vi "Configure Bridge Resistance.vi"(8 "error in (no error)":errorcluster, 9 "Use Rmeas or Ruser (0: Rmeas(System Default Value))":i32(ring) items=["Rmeas(System Default Value)", "Ruser(User Defined Value)"], 10 "Select Bridge Resistance (1: 200Ohm)":i32(ring)=1 items=["100Ohm", "200Ohm", "300Ohm", "400Ohm"], 11 "VISA resource name":refnum<visa-resource-name>) -> (0 "error out":errorcluster, 3 "VISA resource name out":refnum<visa-resource-name>)   [LabVIEW 2011, in "Agilent N432A.lvlib"]
doc: "Specifies the type and value of the bridge resistance for the thermistor sensor. When Rmeas(system default value) is selected, an externally measured bridge resistance value stored in EEPROM will be used. When Ruser(user difined value) is selected, you can enter a resistance value to be used in power measurement."
uses:
  <instrlib>/Agilent N432A/Agilent N432A.lvlib
panel:
  in  "Ruser Value(100 Ohm)":dbl=100.0
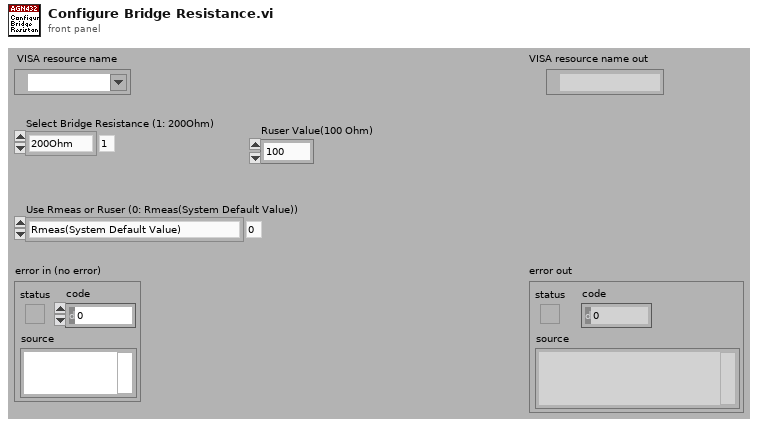
[diagram p1: front panel]
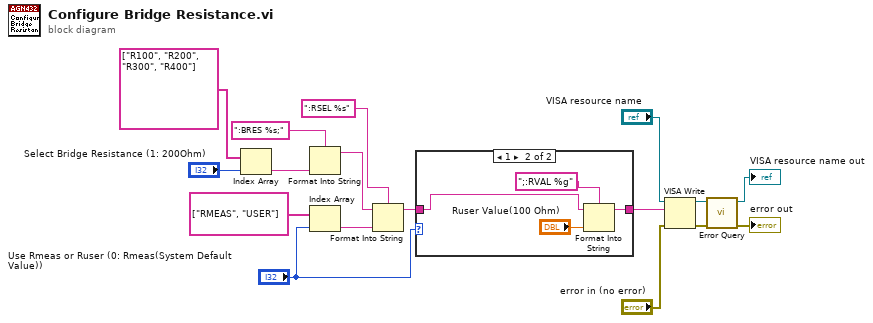
[diagram p0: block diagram]
diagram:
  n1 = Index Array(array=string[] ["R100", "R200", "R300", "R400"], index="Select Bridge Resistance (1: 200Ohm)") -> (element=w6:string)
  n2 = Format Into String(format string=":BRES %s;", w6) -> (resulting string=w3:string)  [unwired: 2 in, 1 out]
  n3 = Index Array(array=string[] ["RMEAS", "USER"], index="Use Rmeas or Ruser (0: Rmeas(System Default Value))") -> (element=w4:string)
  n4 = Format Into String(format string=":RSEL %s", initial string=w3, w4) -> (resulting string=w2:string)  [unwired: 1 in, 1 out]
  n5 = case shown="1" "Use Rmeas or Ruser (0: Rmeas(System Default Value))" {
    tunnel: w2 -> [w18 w20]
    tunnel: [w18 w19] -> w1
    frame 0, Default {
    }
    frame 1 {
      n6 = Format Into String(format string=";:RVAL %g", initial string=w20, "Ruser Value(100 Ohm)") -> (resulting string=w19:string)  [unwired: 1 in, 1 out]
    }
  }
  n7 = VISA Write(VISA resource name="VISA resource name", write buffer=w1, error in (no error)="error in (no error)") -> (VISA resource name out=w15:refnum<visa-resource-name>, error out=w14:errorcluster)  [unwired: 1 out]
  n8 = call <instrlib>:"Error Query.vi"("error in (no error)"=w14, "VISA resource name"=w15) -> ("error out"=→"error out":errorcluster, "VISA resource name out"=→"VISA resource name out":refnum<visa-resource-name>)  [unwired: 6 in, 2 out]
